vi "svfa_Process FRF (1xM).vi"(0 "stimulus signals X [EUx]":waveform(dbl)[](array[waveform]), 1 "response signal Y [EUy]":waveform(dbl), 2 "window":T9=1 items=["None"=0, "Hanning"=1, "Hamming"=2, "Blackman-Harris"=3, "Exact Blackman"=4, "Blackman"=5, "Flat Top"=6, "4 Term B-Harris "=7, "7 Term B-Harris"=8, "Low Sidelobe"=9, "Force - Exponential"=10, "Blackman Nuttall"=11, "Triangle"=30, "Bartlett-Hanning"=31, "Bohman"=32, "Parzen"=33, "Welch"=34, "Kaiser"=60, "Dolph-Chebyshev"=61, "Gaussian"=62], 3 "force/exp settings":T8={"force window [%]"=50.0, "exp window [%]"=10.0} {"exp window [%]" min=0.0 max=100.0 format="%.2f"; "force window [%]" min=0.0 max=100.0 format="%.2f"}, 4 "averaging parameters":T11={"averaging mode"=enum."No averaging", "weighting mode"=enum."Linear", "number of averages"=10, "linear mode"=enum."Auto restart"}, 5 "error in (no error)":errorcluster, 7 "processing control":T10(ring), 9 "FRF mode":enum16{"H1", "H2", "H3"}(ring), 11 "spectra info in":T1[](array[typedef]) {"x-axis units" items=["Time (s)"=0, "Frequency-CB (Hz)"=1, "Frequency-CPB (Hz)"=1248, "Frequency-Arbitrary (Hz)"=2357, "Quefrency (s)"=2, "Revolutions (rev)"=3, "Order"=4, "Speed (RPM)"=11, "Speed (rad/s)"=21, "Index"=65535]; "weighting filter" items=["Linear", "A-weighting", "B-weighting", "C-weighting", "ITU-R 468-4", "Dolby", "CCITT", "C-message", "Wb", "Wc", "Wd", "We", "Wf", "Wh", "Wj", "Wk", "Wm", "AES17 20 kHz lowpass", "AES17 40 kHz lowpass", "AES17 20 kHz highpass", "AES17 40 kHz highpass"]; "dB reference [EU]" format="%.2f"; "engineering units" items=["custom..."=0, "V"=1, "A"=21, "C"=30, "pC"=31, "s"=32, "-"=29, "Pa"=2, "N"=20, "g"=3, "m/s^2"=4, "m/s"=5, "m"=6, "mm/s"=12, "mm"=13, "micron/s"=14, "micron"=15, "in/s^2"=7, "in/s"=8, "in"=9, "mil/s"=10, "mil"=11, "rad/s^2"=16, "rad/s"=17, "rad"=18, "deg/s^2"=26, "deg/s"=27, "deg"=28, "RPM"=22, "cycle/s^2"=23, "Hz"=24, "cycle"=25, "strain"=19]; "spectral info"."window" items=["None "=0, "Hanning"=1, "Hamming"=2, "Blackman-Harris"=3, "Exact Blackman"=4, "Blackman"=5, "Flat Top"=6, "4 Term B-Harris "=7, "7 Term B-Harris"=8, "Low Sidelobe"=9, "Force - Exponential"=10, "Gaussian"=62]}) -> (8 "stimulus signals X [EUx] 2":waveform(dbl)[](array[waveform]), 10 "response signal Y [EUy]":waveform(dbl), 12 "averages completed":dbl format="%.2f", 13 "processing control":T10(ring), 14 "complex responses [EUy/EUx]":T7(array[cluster]) {"complex spectrum" format="%.2f"; "df" format="%.2f"; "f0" format="%.2f"}, 16 "coherence":cluster{"f0":dbl, "df":dbl, "coherence":dbl[]}[](array[cluster]) {"coherence" format="%.2f"; "df" format="%.2f"; "f0" format="%.2f"}, 17 "averaging done":bool, 18 "spectra info out":T1[](array[typedef]) {"x-axis units" items=["Time (s)"=0, "Frequency-CB (Hz)"=1, "Frequency-CPB (Hz)"=1248, "Frequency-Arbitrary (Hz)"=2357, "Quefrency (s)"=2, "Revolutions (rev)"=3, "Order"=4, "Speed (RPM)"=11, "Speed (rad/s)"=21, "Index"=65535]; "weighting filter" items=["Linear", "A-weighting", "B-weighting", "C-weighting", "ITU-R 468-4", "Dolby", "CCITT", "C-message", "Wb", "Wc", "Wd", "We", "Wf", "Wh", "Wj", "Wk", "Wm", "AES17 20 kHz lowpass", "AES17 40 kHz lowpass", "AES17 20 kHz highpass", "AES17 40 kHz highpass"]; "dB reference [EU]" format="%.2f"; "engineering units" items=["custom..."=0, "V"=1, "A"=21, "C"=30, "pC"=31, "s"=32, "-"=29, "Pa"=2, "N"=20, "g"=3, "m/s^2"=4, "m/s"=5, "m"=6, "mm/s"=12, "mm"=13, "micron/s"=14, "micron"=15, "in/s^2"=7, "in/s"=8, "in"=9, "mil/s"=10, "mil"=11, "rad/s^2"=16, "rad/s"=17, "rad"=18, "deg/s^2"=26, "deg/s"=27, "deg"=28, "RPM"=22, "cycle/s^2"=23, "Hz"=24, "cycle"=25, "strain"=19]; "spectral info"."window" items=["None "=0, "Hanning"=1, "Hamming"=2, "Blackman-Harris"=3, "Exact Blackman"=4, "Blackman"=5, "Flat Top"=6, "4 Term B-Harris "=7, "7 Term B-Harris"=8, "Low Sidelobe"=9, "Force - Exponential"=10, "Gaussian"=62]}, 19 "error out":errorcluster)   [LabVIEW 2017]
uses:
  <vilib>/addons/_NISVFA/_Shared subVIs/Controls/svc_Window [Dual FFT].ctl
  <vilib>/addons/_NISVFA/_Shared subVIs/Controls/svc_Spectrum Info.ctl
  <vilib>/addons/_NISVFA/_Shared subVIs/Controls/svc_X-Axis Units.ctl
  <vilib>/addons/_NISVFA/_Shared subVIs/Controls/svc_Spectrum Type.ctl
  <vilib>/addons/_NISVFA/_Shared subVIs/Controls/svc_Engineering Units Text Ring.ctl
  <vilib>/addons/_NISVFA/_Shared subVIs/Controls/svc_Weighting Filter Text Ring.ctl
  <vilib>/addons/_NISVFA/_Shared subVIs/Controls/svc_Complimentary Spectrum Units.ctl
  <vilib>/addons/_NISVFA/_Shared subVIs/Windowing/svfa_Scaled Time Domain Window (N Ch).vi
  <vilib>/addons/_NISVFA/_Shared subVIs/Windowing/svfa_Scaled Time Domain Window (1 Ch).vi
  <vilib>/addons/_NISVFA/_Shared subVIs/Spectrum Averaging/svfa_Average Array (real).vi
  <vilib>/addons/_NISVFA/_Shared subVIs/Spectrum Averaging/svfa_Average Array (complex).vi
  <vilib>/addons/_NISVFA/_Shared subVIs/Windowing/svfa_Scaled Time Domain Window (Array).vi
  <vilib>/Analysis/4window.llb/Force Window.vi
  <vilib>/Analysis/4window.llb/Force Window (DBL).vi
  <vilib>/Analysis/4window.llb/Exponential Window.vi
  <vilib>/Analysis/4window.llb/Exponential Window (DBL).vi
  <vilib>/Utility/error.llb/Error Cluster From Error Code.vi
  <vilib>/Analysis/0measdsp.llb/Scaled Time Domain Window.vi
  <vilib>/Analysis/0measdsp.llb/Scaled Time Domain Window (DBL).vi
  <vilib>/addons/_NISVFA/_Spectrum Processing/subVIs/svfa_Spectrum Info Window to windowTd Type Def.vi
  <vilib>/addons/_NISVFA/_Shared subVIs/Common/svc_Window Parameters.vi
  <vilib>/addons/_NISVFA/_Shared subVIs/Common/svc_Get Window Info.vi
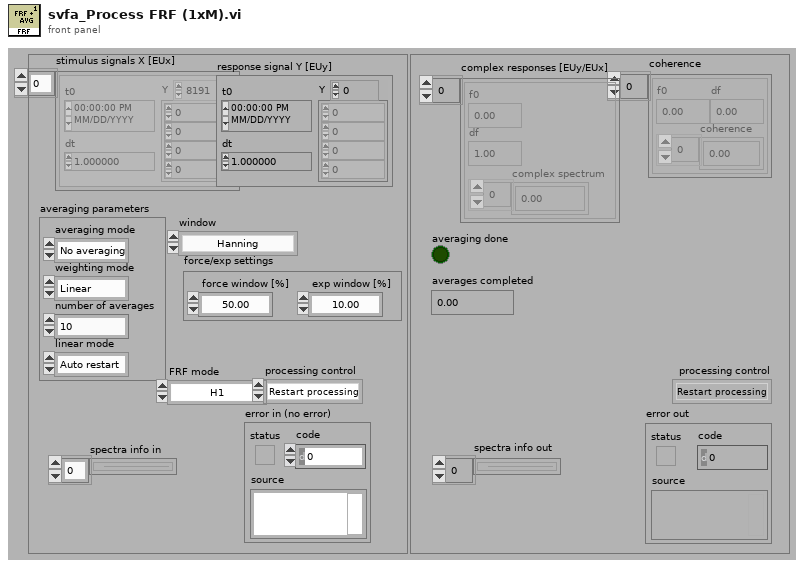
[diagram p1: front panel]
types:
  T1 = typedef "svc_Spectrum Info.ctl" = cluster{"channel name":string, "description":string, "x-axis units":T2, "spectral info":cluster{"spectrum type":T3, "linear/dB":enum16{"linear", "dB"}, "window":u16, "window size":i32, "FFT size":i32}, "engineering units":T4, "custom label":string, "dB reference [EU]":dbl, "peak units":enum16{"rms", "peak", "peak-peak"}, "weighting filter":T5, "spectral density?":bool, "unit label":string, "spectrum skewed?":bool, "complimentary spectrum units":T6}
  T2 = typedef "svc_X-Axis Units.ctl" = u16
  T3 = typedef "svc_Spectrum Type.ctl" = enum16{"FFT Spectrum [complex]", "Amplitude [Magnitude]", "Power [Magnitude^2]", "Cross Spectrum [complex]", "Frequency Response [Complex]"}
  T4 = typedef "svc_Engineering Units Text Ring.ctl" = u16
  T5 = typedef "svc_Weighting Filter Text Ring.ctl" = u16
  T6 = typedef "svc_Complimentary Spectrum Units.ctl" = enum16{"none", "radians", "degrees", "cycles", "imaginary"}
  T7 = cluster{"f0":dbl, "df":dbl, "complex spectrum":cdb[]}[]
  T8 = cluster{"force window [%]":dbl, "exp window [%]":dbl}
  T9 = typedef "svc_Window [Dual FFT].ctl" = u32
  T10 = enum16{"Restart processing", "Continue processing", "Skip processing"}
  T11 = cluster{"averaging mode":enum16{"No averaging", "Vector averaging", "RMS averaging", "Peak hold"}, "weighting mode":enum16{"Linear", "Exponential"}, "number of averages":u32, "linear mode":enum16{"One shot", "Auto restart"}}
  T12 = enum16{"No averaging", "Vector averaging", "RMS averaging", "Peak hold"}
  T13 = cluster{"f0":dbl, "df":dbl, "complex array":cdb[]}
  T14 = cluster{"f0":dbl, "df":dbl, "complex array":cdb[]}[]
  T15 = cluster{"complex spectrum":cluster{"f0":dbl, "df":dbl, "complex spectrum":cdb[]}, "spectrum info":T1}
  T16 = cluster{"f0":dbl, "df":dbl, "complex spectrum":cdb[]}
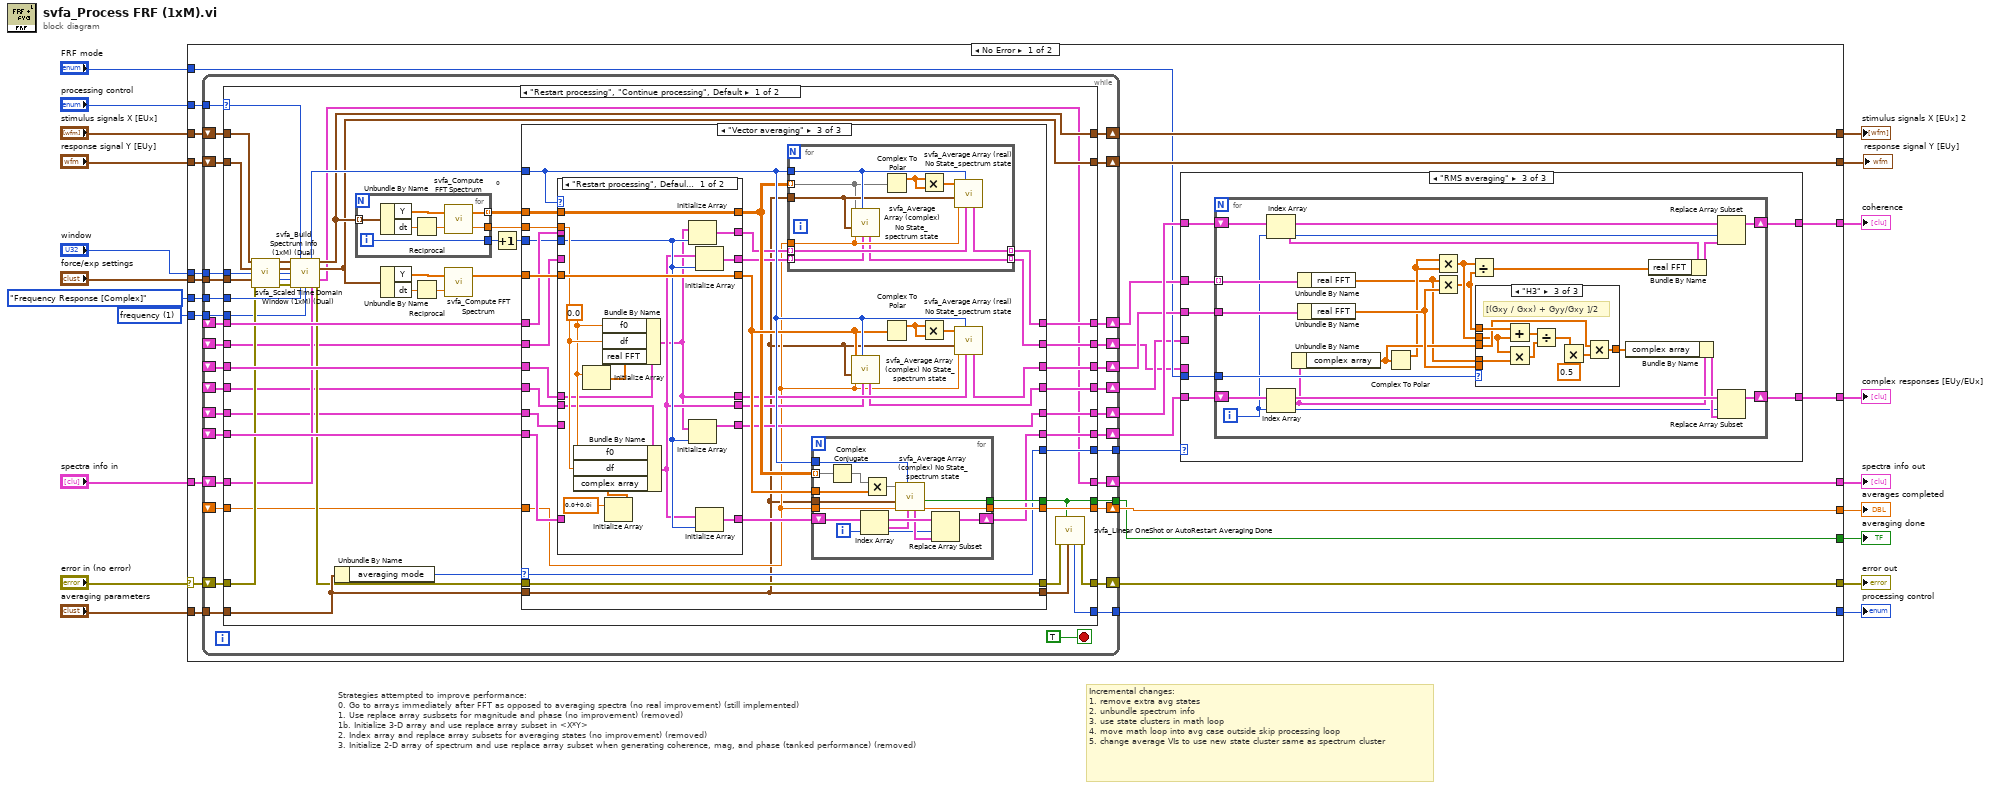
[diagram p0: block diagram]
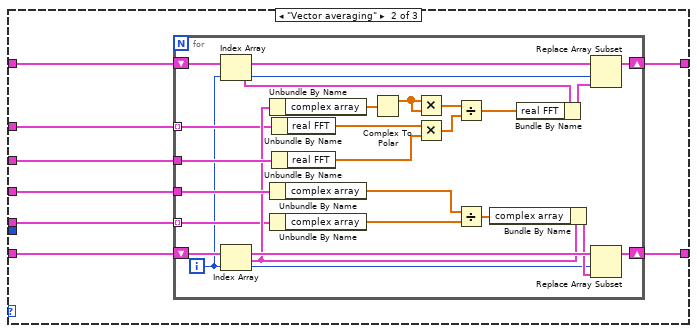
[diagram p3: hidden frame]
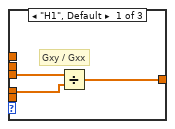
[diagram p4: hidden frame]
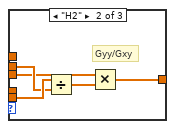
[diagram p5: hidden frame]
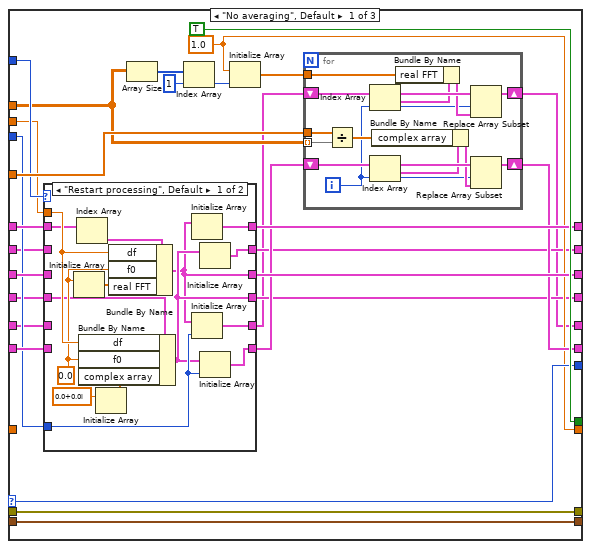
[diagram p6: hidden frame]
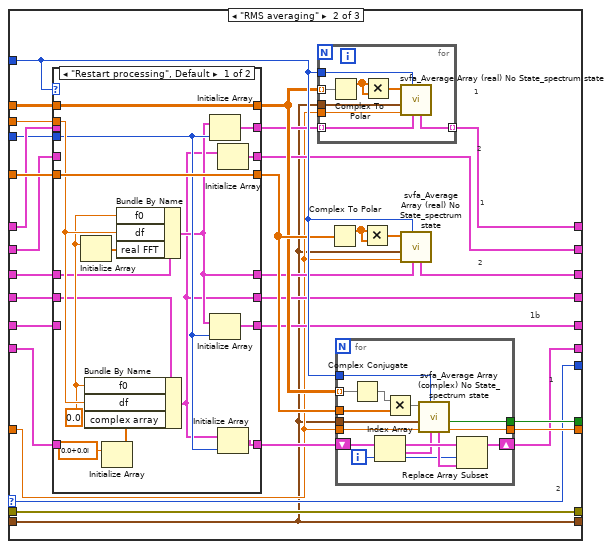
[diagram p8: hidden frame]
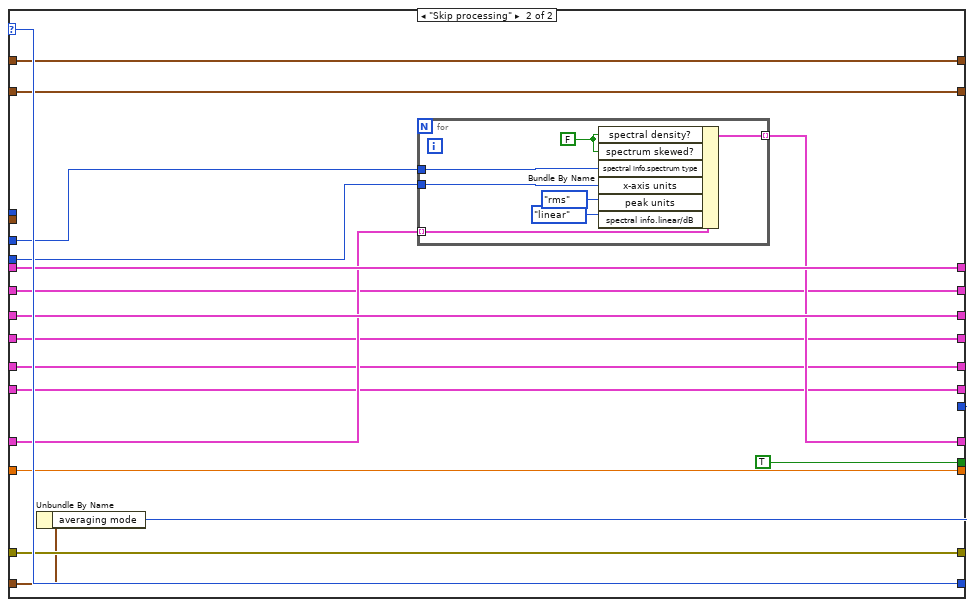
[diagram p11: hidden frame]
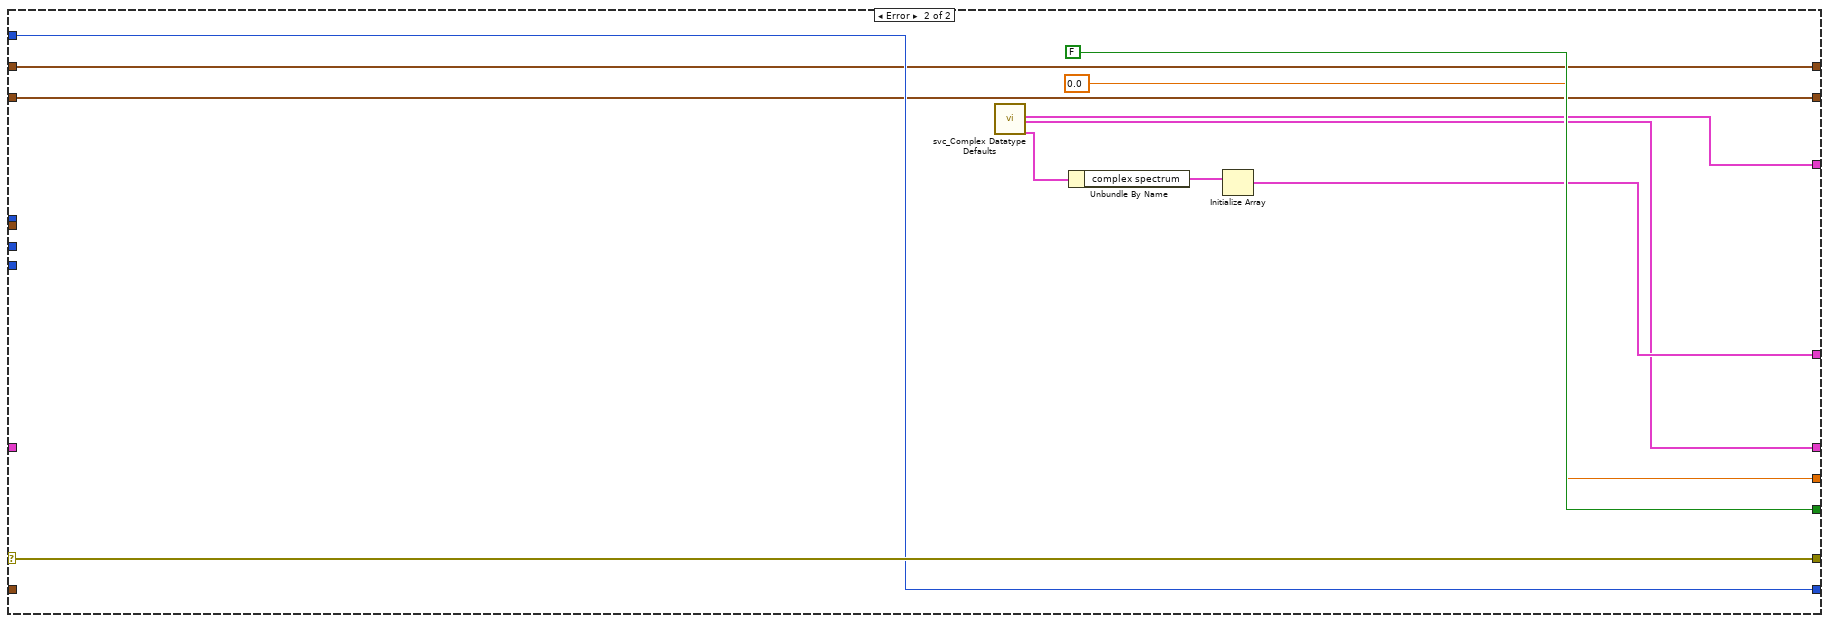
[diagram p12: hidden frame]
diagram:
  w6 = u16 1 items=["time"=0, "frequency"=1, "quefrency"=2, "revolutions"=3, "order"=4, "rpm"=11] ("x-axis units")
  # "Strategies attempted to improve performance:\n0. Go to arrays immediately after FFT as opposed to averaging spectra (no real improvement) (still implemented)\n1. Use replace array susbsets for magnitude and phase (no improvement) (removed)\n1b. Initialize 3-D array and use replace array subset in <X*Y>\n2. Index array and replace array subsets for averaging states (no improvement) (removed)\n3. Initialize 2-D array of spectrum and use replace array subset when generating coherence, mag, and phase (tanked performance) (removed)"
  # "Incremental changes:\n1. remove extra avg states\n2. unbundle spectrum info\n3. use state clusters in math loop\n4. move math loop into avg case outside skip processing loop\n5. change average VIs to use new state cluster same as spectrum cluster"
  n1 = case shown="No Error" "error in (no error)" {
    selector: "error in (no error)" -> [w44 w467]
    tunnel: [w38 w467] -> w20
    tunnel: "averaging parameters" -> [w47 _]
    tunnel: "stimulus signals X [EUx]" -> [w45 w460]
    tunnel: [w32 FALSE ("averaging done")] -> w16
    tunnel: [w46 0.0 ("averages completed")] -> w15
    tunnel: [w22 w461] -> w14
    tunnel: [w23 w457] -> w13
    tunnel: "FRF mode" -> [w26 _]
    tunnel: "processing control" -> [w43 w464]
    tunnel: [w39 w464] -> w10
    tunnel: "response signal Y [EUy]" -> [w42 w459]
    tunnel: "window" -> [w41 _]
    tunnel: "force/exp settings" -> [w40 _]
    tunnel: svc_Spectrum_Type."Frequency Response [Complex]" ("spectrum type") -> [w37 _]
    tunnel: w6 -> [w36 _]
    tunnel: [w35 w458] -> w5
    tunnel: [w34 w460] -> w4
    tunnel: [w33 w459] -> w3
    tunnel: "spectra info in" -> [w21 _]
    frame No Error {
      n2 = while {
        tunnel: [w149] -> w39
        tunnel: w40 -> [w150]
        tunnel: w41 -> [w151]
        tunnel: w43 -> [w146]
        tunnel: [w155] -> w32
        tunnel: w47 -> [w157]
        shift-right: [w145] -> w28
        shift-left: _ -> [w144]
        shift-right: [w127] -> w31
        shift-left: _ -> [w130]
        shift-right: [w143] -> w29
        shift-left: _ -> [w142]
        tunnel: w37 -> [w141]
        tunnel: w36 -> [w140]
        tunnel: [w137] -> w27
        shift-right: [w136] -> w34
        shift-left: w45 -> [w154]
        shift-right: [w135] -> w33
        shift-left: w42 -> [w152]
        shift-right: [w148] -> w38
        shift-left: w44 -> [w153]
        shift-right: [w138] -> w35
        shift-left: w21 -> [w139]
        shift-right: [w129] -> w24
        shift-left: _ -> [w132]
        shift-right: [w128] -> w25
        shift-left: _ -> [w131]
        shift-right: [w134] -> w30
        shift-left: _ -> [w133]
        shift-right: [w156] -> w46
        shift-left: _ -> [w126]
        stop <- TRUE stop-if-true
        n3 = case shown="\"Restart processing\", \"Continue processing\", Default" w146 {
          selector: w146 -> [w158 w449]
          tunnel: w157 -> [w193 w440]
          tunnel: [w205 w436] -> w156
          tunnel: [w204 TRUE ("averaging done")] -> w155
          tunnel: w153 -> [w179 w447]
          tunnel: w152 -> [w200 w437]
          tunnel: w151 -> [w199 _]
          tunnel: w150 -> [w189 _]
          tunnel: [w196 w449] -> w149
          tunnel: [w194 w447] -> w148
          tunnel: w154 -> [w201 w438]
          tunnel: [w188 w441] -> w134
          tunnel: [w187 w446] -> w145
          tunnel: w133 -> [w186 w441]
          tunnel: w144 -> [w185 w446]
          tunnel: [w184 w445] -> w143
          tunnel: w142 -> [w183 w445]
          tunnel: w141 -> [w182 w432]
          tunnel: w140 -> [w176 w442]
          tunnel: w139 -> [w175 w444]
          tunnel: [w159 w443] -> w138
          tunnel: [w174 w439] -> w137
          tunnel: [w171 w438] -> w136
          tunnel: [w170 w437] -> w135
          tunnel: w132 -> [w169 w435]
          tunnel: w131 -> [w168 w434]
          tunnel: w130 -> [w167 w433]
          tunnel: [w166 w435] -> w129
          tunnel: [w165 w434] -> w128
          tunnel: [w164 w433] -> w127
          tunnel: w126 -> [w163 w436]
          frame "Restart processing", "Continue processing", Default {
            # "0"
            n4 = call <vilib>:"svfa_Scaled Time Domain Window (1xM) (Dual).vi"("stimulus signals X [EUx]"=w201, "response signal Y [EUy]"=w200, "window"=w199, "force and exponential window settings"=w189, "error in (no error)"=w179) -> ("stimulus signals X [EUx]"=w203:waveform(dbl)[], "response signal Y [EUy]"=w202:waveform(dbl), "window"=w198:u16, "window size"=w191:i32, "error out"=w190:errorcluster)  [unwired: 6 in]
            n5 = call <vilib>:"svfa_Build Spectrum Info (1xM) (Dual).vi"("stimulus signals X [EUx]"=w203, "processing control"=w158, "response signal Y [EUy]"=w202, "window"=w198, "window size"=w191, "error in (no error)"=w190, "spectrum type"=w182, "x-axis units"=w176, "spectra info in"=w175) -> ("dup processing control"=w195:T10, "dup stimulus signals X [EUx]"=w171:waveform(dbl)[], "response signal Y [EUy]"=w170:waveform(dbl), "spectra info out"=w159:T1[], "error out"=w172:errorcluster)  [unwired: 2 in]
            n6 = Unbundle By Name(w193) -> ("averaging mode"=w206:T12)
            n7 = for {
              tunnel: w171 -> [w213] mode=indexing
              tunnel: [w209] -> w192 mode=indexing
              tunnel: [w208] -> w173
              tunnel: [w207] -> w178
              i -> [w207]
              n8 = Unbundle By Name ("Get Waveform Components")(w213) -> ("Y"=w212:dbl[], "dt"=w211:dbl)
              n9 = Reciprocal(x=w211) -> (1/x=w210:dbl)
              n10 = call <vilib>:"svfa_Compute FFT Spectrum.vi"("sampling frequency [Hz]"=w210, "signal [EU]"=w212) -> ("df [Hz]"=w208:dbl, "FFT spectrum [EUrms]"=w209:cdb[])
            }
            n11 = Unbundle By Name ("Get Waveform Components")(w170) -> ("Y"=w162:dbl[], "dt"=w161:dbl)
            n12 = Reciprocal(x=w161) -> (1/x=w160:dbl)
            n13 = call <vilib>:"svfa_Compute FFT Spectrum.vi"("sampling frequency [Hz]"=w160, "signal [EU]"=w162) -> ("FFT spectrum [EUrms]"=w181:cdb[])  [unwired: 1 out]
            n14 = Increment(x=w178) -> (x+1=w177:i32)
            n15 = case shown="\"Vector averaging\"" w206 {
              selector: w206 -> [w228 w288 w365]
              tunnel: [w239 w287 w364] -> w180
              tunnel: w172 -> [w239 w287 w364]
              tunnel: w193 -> [w240 w279 w354]
              tunnel: [TRUE ("averaging done") w305 w383] -> w204
              tunnel: w195 -> [w237 w303 w381]
              tunnel: [w223 w304 w382] -> w205
              tunnel: [w240 w279 w354] -> w197
              tunnel: w192 -> [w226 w301 w379]
              tunnel: w181 -> [w238 w302 w380]
              tunnel: [w229 w292 w366] -> w188
              tunnel: [w232 w290 w368] -> w187
              tunnel: w186 -> [w234 w295 w374]
              tunnel: w185 -> [w235 w294 w371]
              tunnel: [w233 w291 w369] -> w184
              tunnel: w183 -> [w236 w293 w372]
              tunnel: w173 -> [w227 w289 w367]
              tunnel: w177 -> [w231 w278 w370]
              tunnel: [w228 w288 w365] -> w174
              tunnel: w169 -> [w217 w285 w358]
              tunnel: w168 -> [w219 w283 w357]
              tunnel: w167 -> [w220 w281 w356]
              tunnel: [w218 w286 w362] -> w166
              tunnel: [w216 w284 w360] -> w165
              tunnel: [w214 w282 w359] -> w164
              tunnel: w163 -> [_ w280 w355]
              frame "No averaging", Default {
                w223 = 1.0 ("overwrite value")
                n16 = case shown="\"Restart processing\", Default" w237 {
                  tunnel: [w265 w275] -> w233
                  tunnel: w236 -> [w263 w275]
                  tunnel: [w255 w274] -> w232
                  tunnel: w235 -> [_ w274]
                  tunnel: [w269 w273] -> w230
                  tunnel: w234 -> [_ w273]
                  tunnel: w231 -> [w266 _]
                  tunnel: w227 -> [w268 _]
                  tunnel: w220 -> [_ w270]
                  tunnel: w219 -> [w257 w271]
                  tunnel: w217 -> [_ w272]
                  tunnel: [w264 w272] -> w218
                  tunnel: [w256 w271] -> w216
                  tunnel: [w267 w270] -> w215
                  frame "Restart processing", Default {
                    w261 = 0.0 ("f0")
                    n17 = Initialize Array(w261) -> (w262:dbl[])  [unwired: 1 in]
                    n18 = Index Array(array=w263) -> (element=w258:cluster{"f0":dbl, "df":dbl, "real FFT":dbl[]})  [unwired: 1 in]
                    n19 = Initialize Array(cdb 0.0+0.0i ("element")) -> (w259:cdb[])  [unwired: 1 in]
                    n20 = Bundle By Name(cluster=w257, "df"=w268, "f0"=w261, "complex array"=w259) -> (w256:T13)
                    n21 = Bundle By Name(cluster=w258, "df"=w268, "f0"=w261, "real FFT"=w262) -> (w255:cluster{"f0":dbl, "df":dbl, "real FFT":dbl[]})
                    n22 = Initialize Array(w255) -> (w265:cluster{"f0":dbl, "df":dbl, "real FFT":dbl[]}[])  [unwired: 1 in]
                    n23 = Initialize Array(w255, w266) -> (w267:cluster{"f0":dbl, "df":dbl, "real FFT":dbl[]}[])
                    n24 = Initialize Array(w256) -> (w264:T14)  [unwired: 1 in]
                    n25 = Initialize Array(w256, w266) -> (w269:T14)
                  }
                  frame "Continue processing" {
                  }
                }
                n26 = Array Size(array=w226) -> (size(s)=w225:i32[])
                n27 = Index Array(array=w225, index=1) -> (element=w224:i32)
                n28 = Initialize Array(w223, w224) -> (w222:dbl[])
                n29 = for {
                  tunnel: w222 -> [w246]
                  tunnel: w226 -> [w248] mode=indexing
                  tunnel: w238 -> [w254]
                  shift-right: [w251] -> w229
                  shift-left: w230 -> [w252]
                  shift-right: [w243] -> w214
                  shift-left: w215 -> [w247]
                  i -> [w242]
                  n30 = Divide(x=w254, y=w248) -> (x/y=w253:cdb[])
                  n31 = Index Array(array=w247, index=w242) -> (element=w245:cluster{"f0":dbl, "df":dbl, "real FFT":dbl[]})
                  n32 = Index Array(array=w252, index=w242) -> (element=w249:T13)
                  n33 = Bundle By Name(cluster=w249, "complex array"=w253) -> (w250:T13)
                  n34 = Bundle By Name(cluster=w245, "real FFT"=w246) -> (w244:cluster{"f0":dbl, "df":dbl, "real FFT":dbl[]})
                  n35 = Replace Array Subset(array=w247, new element=w244, index=w242) -> (w243:cluster{"f0":dbl, "df":dbl, "real FFT":dbl[]}[])
                  n36 = Replace Array Subset(array=w252, new element=w250, index=w242) -> (w251:T14)
                }
              }
              frame "RMS averaging" {
                # "1"
                # "1b"
                # "2"
                # "2"
                # "2"
                # "1"
                # "1"
                n37 = case shown="\"Restart processing\", Default" w303 {
                  tunnel: w302 -> [w335 w340]
                  tunnel: w301 -> [w329 w343]
                  tunnel: [w335 w340] -> w300
                  tunnel: [w329 w343] -> w299
                  tunnel: [w334 w342] -> w298
                  tunnel: [w333 w341] -> w297
                  tunnel: [w323 w339] -> w296
                  tunnel: w295 -> [_ w342]
                  tunnel: w293 -> [_ w341]
                  tunnel: w294 -> [w322 w339]
                  tunnel: w278 -> [w328 _]
                  tunnel: w289 -> [w332 _]
                  tunnel: [w331 w338] -> w286
                  tunnel: w285 -> [_ w338]
                  tunnel: [w320 w337] -> w284
                  tunnel: w283 -> [w321 w337]
                  tunnel: [w330 w336] -> w282
                  tunnel: w281 -> [_ w336]
                  frame "Restart processing", Default {
                    w326 = 0.0 ("f0")
                    n38 = Initialize Array(w326) -> (w327:dbl[])  [unwired: 1 in]
                    n39 = Initialize Array(cdb 0.0+0.0i ("element")) -> (w324:cdb[])  [unwired: 1 in]
                    n40 = Bundle By Name(cluster=w321, "f0"=w326, "df"=w332, "complex array"=w324) -> (w320:T13)
                    n41 = Bundle By Name(cluster=w322, "f0"=w326, "df"=w332, "real FFT"=w327) -> (w323:cluster{"f0":dbl, "df":dbl, "real FFT":dbl[]})
                    n42 = Initialize Array(w323, w328) -> (w333:cluster{"f0":dbl, "df":dbl, "real FFT":dbl[]}[])
                    n43 = Initialize Array(w323, w328) -> (w330:cluster{"f0":dbl, "df":dbl, "real FFT":dbl[]}[])
                    n44 = Initialize Array(w320) -> (w331:T14)  [unwired: 1 in]
                    n45 = Initialize Array(w320, w328) -> (w334:T14)
                  }
                  frame "Continue processing", "Skip processing" {
                  }
                }
                n46 = for {
                  tunnel: w299 -> [w348] mode=indexing
                  tunnel: w303 -> [w351]
                  tunnel: w280 -> [w346]
                  tunnel: w297 -> [w344] mode=indexing
                  tunnel: [w345] -> w291 mode=indexing
                  tunnel: w279 -> [w347]
                  n47 = Complex To Polar(r * e^(i*theta)=w348) -> (r=w350:dbl[])  [unwired: 1 out]
                  n48 = Multiply(x=w350, y=w350) -> (x*y=w349:dbl[])
                  n49 = call <vilib>:"svfa_Average Array (real) No State_spectrum state.vi"("previous avg real spectrum"=w344, "processing control"=w351, "averages completed"=w346, "averaging parameters"=w347, "array"=w349) -> ("new avg real spectrum"=w345:cluster{"f0":dbl, "df":dbl, "real FFT":dbl[]})  [unwired: 4 in, 2 out]
                }
                n50 = Complex To Polar(r * e^(i*theta)=w300) -> (r=w277:dbl[])  [unwired: 1 out]
                n51 = for {
                  tunnel: w303 -> [w317]
                  tunnel: w279 -> [w319]
                  tunnel: w300 -> [w314]
                  tunnel: [w316] -> w305
                  tunnel: [w315] -> w304
                  shift-right: [w312] -> w292
                  shift-left: w298 -> [w313]
                  tunnel: w280 -> [w309]
                  tunnel: w299 -> [w307] mode=indexing
                  i -> [w306]
                  n52 = Complex Conjugate(1:w307) -> (0:w308:cdb[])
                  n53 = Index Array(array=w313, index=w306) -> (element=w310:T13)
                  n54 = Multiply(x=w308, y=w314) -> (x*y=w318:cdb[])
                  n55 = call <vilib>:"svfa_Average Array (complex) No State_spectrum state.vi"("previous avg complex spectrum"=w310, "processing control"=w317, "averages completed in"=w309, "averaging parameters"=w319, "array"=w318) -> ("averages completed out"=w315:dbl, "averaging done"=w316:bool, "avg complex spectrum"=w311:T13)  [unwired: 4 in]
                  n56 = Replace Array Subset(array=w313, new element=w311, index=w306) -> (w312:T14)
                }
                n57 = Multiply(x=w277, y=w277) -> (x*y=w276:dbl[])
                n58 = call <vilib>:"svfa_Average Array (real) No State_spectrum state.vi"("previous avg real spectrum"=w296, "processing control"=w303, "averages completed"=w280, "averaging parameters"=w279, "array"=w276) -> ("new avg real spectrum"=w290:cluster{"f0":dbl, "df":dbl, "real FFT":dbl[]})  [unwired: 4 in, 2 out]
              }
              frame "Vector averaging" {
                n59 = case shown="\"Restart processing\", Default" w381 {
                  tunnel: w380 -> [w413 w421]
                  tunnel: w379 -> [w407 w420]
                  tunnel: [w413 w421] -> w378
                  tunnel: [w407 w420] -> w377
                  tunnel: [w412 w419] -> w376
                  tunnel: [w411 w418] -> w375
                  tunnel: w374 -> [_ w419]
                  tunnel: w372 -> [_ w418]
                  tunnel: [w398 w417] -> w373
                  tunnel: w371 -> [w401 w417]
                  tunnel: w370 -> [w406 _]
                  tunnel: w367 -> [w408 _]
                  tunnel: [w410 w416] -> w363
                  tunnel: [w399 w415] -> w361
                  tunnel: [w409 w414] -> w359
                  tunnel: w358 -> [_ w416]
                  tunnel: w357 -> [w400 w415]
                  tunnel: w356 -> [_ w414]
                  frame "Restart processing", Default {
                    w405 = 0.0 ("f0")
                    n60 = Initialize Array(w405) -> (w404:dbl[])  [unwired: 1 in]
                    n61 = Bundle By Name(cluster=w401, "f0"=w405, "df"=w408, "real FFT"=w404) -> (w398:cluster{"f0":dbl, "df":dbl, "real FFT":dbl[]})
                    n62 = Initialize Array(cdb 0.0+0.0i ("element")) -> (w402:cdb[])  [unwired: 1 in]
                    n63 = Bundle By Name(cluster=w400, "f0"=w405, "df"=w408, "complex array"=w402) -> (w399:T13)
                    n64 = Initialize Array(w398, w406) -> (w411:cluster{"f0":dbl, "df":dbl, "real FFT":dbl[]}[])
                    n65 = Initialize Array(w398, w406) -> (w409:cluster{"f0":dbl, "df":dbl, "real FFT":dbl[]}[])
                    n66 = Initialize Array(w399, w406) -> (w410:T14)
                    n67 = Initialize Array(w399, w406) -> (w412:T14)
                  }
                  frame "Continue processing", "Skip processing" {
                  }
                }
                n68 = for {
                  tunnel: w377 -> [w422] mode=indexing
                  tunnel: w381 -> [w431]
                  tunnel: w375 -> [w427] mode=indexing
                  tunnel: [w426] -> w369 mode=indexing
                  tunnel: w363 -> [w424] mode=indexing
                  tunnel: [w423] -> w362 mode=indexing
                  tunnel: w355 -> [w428]
                  tunnel: w354 -> [w425]
                  n69 = call <vilib>:"svfa_Average Array (complex) No State_spectrum state.vi"("previous avg complex spectrum"=w424, "processing control"=w431, "averages completed in"=w428, "averaging parameters"=w425, "array"=w422) -> ("avg complex spectrum"=w423:T13)  [unwired: 4 in, 2 out]
                  n70 = Complex To Polar(r * e^(i*theta)=w422) -> (r=w430:dbl[])  [unwired: 1 out]
                  n71 = Multiply(x=w430, y=w430) -> (x*y=w429:dbl[])
                  n72 = call <vilib>:"svfa_Average Array (real) No State_spectrum state.vi"("previous avg real spectrum"=w427, "processing control"=w431, "averages completed"=w428, "averaging parameters"=w425, "array"=w429) -> ("new avg real spectrum"=w426:cluster{"f0":dbl, "df":dbl, "real FFT":dbl[]})  [unwired: 4 in, 2 out]
                }
                n73 = for {
                  tunnel: w381 -> [w395]
                  tunnel: w354 -> [w392]
                  tunnel: w377 -> [w391] mode=indexing
                  tunnel: w378 -> [w390]
                  tunnel: [w394] -> w383
                  tunnel: [w393] -> w382
                  shift-right: [w386] -> w366
                  shift-left: w376 -> [w389]
                  tunnel: w355 -> [w385]
                  i -> [w384]
                  n74 = Complex Conjugate(1:w391) -> (0:w397:cdb[])
                  n75 = Index Array(array=w389, index=w384) -> (element=w387:T13)
                  n76 = Multiply(x=w397, y=w390) -> (x*y=w396:cdb[])
                  n77 = call <vilib>:"svfa_Average Array (complex) No State_spectrum state.vi"("previous avg complex spectrum"=w387, "processing control"=w395, "averages completed in"=w385, "averaging parameters"=w392, "array"=w396) -> ("averages completed out"=w393:dbl, "averaging done"=w394:bool, "avg complex spectrum"=w388:T13)  [unwired: 4 in]
                  n78 = Replace Array Subset(array=w389, new element=w388, index=w384) -> (w386:T14)
                }
                n79 = call <vilib>:"svfa_Average Array (complex) No State_spectrum state.vi"("previous avg complex spectrum"=w361, "processing control"=w381, "averages completed in"=w355, "averaging parameters"=w354, "array"=w378) -> ("avg complex spectrum"=w360:T13)  [unwired: 4 in, 2 out]
                n80 = Complex To Polar(r * e^(i*theta)=w378) -> (r=w353:dbl[])  [unwired: 1 out]
                n81 = Multiply(x=w353, y=w353) -> (x*y=w352:dbl[])
                n82 = call <vilib>:"svfa_Average Array (real) No State_spectrum state.vi"("previous avg real spectrum"=w373, "processing control"=w381, "averages completed"=w355, "averaging parameters"=w354, "array"=w352) -> ("new avg real spectrum"=w368:cluster{"f0":dbl, "df":dbl, "real FFT":dbl[]})  [unwired: 4 in, 2 out]
              }
            }
            n83 = call <vilib>:"svfa_Linear OneShot or AutoRestart Averaging Done.vi"("averaging parameters"=w197, "averaging done"=w204, "error in (no error)"=w180) -> ("error out"=w194:errorcluster, "processing control"=w196:T10)  [unwired: 7 in]
          }
          frame "Skip processing" {
            n84 = Unbundle By Name(w440) -> ("averaging mode"=w439:T12)
            n85 = for {
              tunnel: w444 -> [w453] mode=indexing
              tunnel: [w452] -> w443 mode=indexing
              tunnel: w432 -> [w451]
              tunnel: w442 -> [w450]
              w455 = FALSE ("spectral density?")
              n86 = Bundle By Name(cluster=w453, "spectral density?"=w455, "spectrum skewed?"=w455, "spectral info.spectrum type"=w451, "x-axis units"=w450, "peak units"=enum16{"rms", "peak", "peak-peak"}."rms", "spectral info.linear/dB"=enum16{"linear", "dB"}."linear") -> (w452:T1)
            }
          }
        }
      }
      n87 = case shown="\"RMS averaging\"" w27 {
        tunnel: w30 -> [w48 w57 w85]
        tunnel: w28 -> [_ w56 w86]
        tunnel: w29 -> [_ w55 w87]
        tunnel: [w49 w51 w83] -> w23
        tunnel: [w48 w50 w84] -> w22
        tunnel: w26 -> [_ _ w82]
        tunnel: w31 -> [w49 w52 w81]
        tunnel: w24 -> [_ w54 _]
        tunnel: w25 -> [_ w53 _]
        frame "No averaging", Default {
        }
        frame "Vector averaging" {
          n88 = for {
            tunnel: w55 -> [w62] mode=indexing
            tunnel: w56 -> [w78]
            tunnel: w53 -> [w75]
            tunnel: w54 -> [w59] mode=indexing
            shift-right: [w67] -> w51
            shift-left: w52 -> [w71]
            shift-right: [w72] -> w50
            shift-left: w57 -> [w73]
            i -> [w58]
            n89 = Index Array(array=w71, index=w58) -> (element=w70:cluster{"f0":dbl, "df":dbl, "real FFT":dbl[]})
            n90 = Index Array(array=w73, index=w58) -> (element=w65:T13)
            n91 = Unbundle By Name(w65) -> ("complex array"=w76:cdb[])
            n92 = Unbundle By Name(w75) -> ("complex array"=w74:cdb[])
            n93 = Unbundle By Name(w59) -> ("complex array"=w60:cdb[])
            n94 = Unbundle By Name(w62) -> ("real FFT"=w61:dbl[])
            n95 = Unbundle By Name(w78) -> ("real FFT"=w77:dbl[])
            n96 = Complex To Polar(r * e^(i*theta)=w76) -> (r=w63:dbl[])  [unwired: 1 out]
            n97 = Multiply(x=w63, y=w63) -> (x*y=w80:dbl[])
            n98 = Multiply(x=w61, y=w77) -> (x*y=w79:dbl[])
            n99 = Divide(x=w80, y=w79) -> (x/y=w68:dbl[])
            n100 = Divide(x=w74, y=w60) -> (x/y=w64:cdb[])
            n101 = Bundle By Name(cluster=w65, "complex array"=w64) -> (w66:T13)
            n102 = Bundle By Name(cluster=w70, "real FFT"=w68) -> (w69:cluster{"f0":dbl, "df":dbl, "real FFT":dbl[]})
            n103 = Replace Array Subset(array=w71, new element=w69, index=w58) -> (w67:cluster{"f0":dbl, "df":dbl, "real FFT":dbl[]}[])
            n104 = Replace Array Subset(array=w73, new element=w66, index=w58) -> (w72:T14)
          }
        }
        frame "RMS averaging" {
          n105 = for {
            tunnel: w87 -> [w90] mode=indexing
            tunnel: w86 -> [w107]
            tunnel: w82 -> [w106]
            shift-right: [w103] -> w83
            shift-left: w81 -> [w104]
            shift-right: [w97] -> w84
            shift-left: w85 -> [w99]
            i -> [w88]
            n106 = Index Array(array=w104, index=w88) -> (element=w102:cluster{"f0":dbl, "df":dbl, "real FFT":dbl[]})
            n107 = Index Array(array=w99, index=w88) -> (element=w96:T13)
            n108 = Unbundle By Name(w96) -> ("complex array"=w95:cdb[])
            n109 = Unbundle By Name(w90) -> ("real FFT"=w91:dbl[])
            n110 = Unbundle By Name(w107) -> ("real FFT"=w105:dbl[])
            n111 = Complex To Polar(r * e^(i*theta)=w95) -> (r=w92:dbl[])  [unwired: 1 out]
            n112 = Multiply(x=w92, y=w92) -> (x*y=w93:dbl[])
            n113 = Multiply(x=w91, y=w105) -> (x*y=w89:dbl[])
            n114 = Divide(x=w93, y=w89) -> (x/y=w101:dbl[])
            n115 = case shown="\"H3\"" w106 {
              tunnel: [w110 w111 w123] -> w94
              tunnel: w91 -> [w109 _ w119]
              tunnel: w105 -> [_ w115 _]
              tunnel: w95 -> [w108 w112 w117]
              tunnel: w93 -> [_ w114 w116]
              tunnel: w89 -> [_ _ w122]
              frame "H1", Default {
                # "Gxy / Gxx"
                n116 = Divide(x=w108, y=w109) -> (x/y=w110:cdb[])
              }
              frame "H2" {
                # "Gyy/Gxy"
                n117 = Divide(x=w115, y=w114) -> (x/y=w113:dbl[])
                n118 = Multiply(x=w112, y=w113) -> (x*y=w111:cdb[])
              }
              frame "H3" {
                # "[(Gxy / Gxx) + Gyy/Gxy ]/2"
                n119 = Add(x=w122, y=w116) -> (x+y=w121:dbl[])
                n120 = Multiply(x=w116, y=w119) -> (x*y=w118:dbl[])
                n121 = Divide(x=w121, y=w118) -> (x/y=w120:dbl[])
                n122 = Multiply(x=w120, y=0.5) -> (x*y=w124:dbl[])
                n123 = Multiply(x=w117, y=w124) -> (x*y=w123:cdb[])
              }
            }
            n124 = Bundle By Name(cluster=w96, "complex array"=w94) -> (w98:T13)
            n125 = Bundle By Name(cluster=w102, "real FFT"=w101) -> (w100:cluster{"f0":dbl, "df":dbl, "real FFT":dbl[]})
            n126 = Replace Array Subset(array=w104, new element=w100, index=w88) -> (w103:cluster{"f0":dbl, "df":dbl, "real FFT":dbl[]}[])
            n127 = Replace Array Subset(array=w99, new element=w98, index=w88) -> (w97:T14)
          }
        }
      }
    }
    frame Error {
      n128 = call <vilib>:"svc_Complex Datatype Defaults.vi"() -> ("empty array of spectra"=w457:cluster{"f0":dbl, "df":dbl, "magnitude":dbl[]}[], "empty array of spectrum info"=w458:T1[], "complex spectrum"=w463:T15)  [unwired: 11 in, 6 out]
      n129 = Unbundle By Name(w463) -> ("complex spectrum"=w462:T16)
      n130 = Initialize Array(w462) -> (w461:T7)  [unwired: 1 in]
    }
  }
  "error out" <- w20
  "averages completed" <- w15
  "averaging done" <- w16
  "complex responses [EUy/EUx]" <- w14
  "coherence" <- w13
  "processing control" <- w10
  "spectra info out" <- w5
  "stimulus signals X [EUx] 2" <- w4
  "response signal Y [EUy]" <- w3
